vi "Test Upload to S3.vi"() -> ()   [LabVIEW 2016, in "Control Experiment.lvclass"]
uses:
  Control Experiment.lvclass
panel:
  in  "file to upload":path
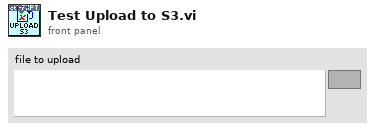
[diagram p1: front panel]
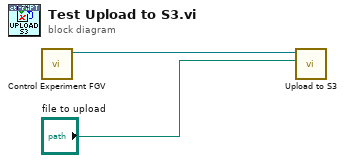
[diagram p0: block diagram]
diagram:
  n1 = call "Control Experiment FGV.vi"() -> ("Control Experiment.lvclass out"=w1:refnum<class "Control Experiment.lvclass">)  [unwired: 10 in, 1 out]
  n2 = call "Upload to S3.vi"(10:"file to upload", "Control Experiment in"=w1) -> ()  [unwired: 9 in, 1 out]
